vi "Recursive path search.vi"(6 "File name with extension":string, 8 "error in":errorcluster, 11 "Path":path) -> (0 "error out":errorcluster, 3 "Path out":path)   [LabVIEW 2019, in "TDMS.lvlib" / "TDMS.lvclass"]
uses:
  TDMS.lvclass
  <vilib>/Utility/sysdir.llb/System Directory Type.ctl
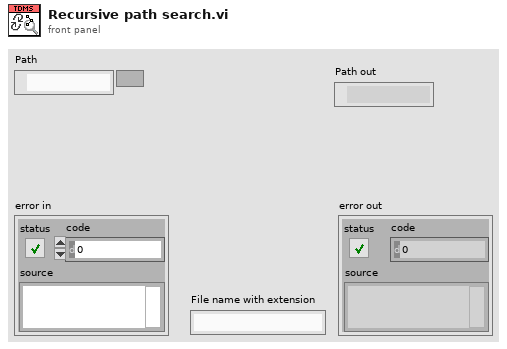
[diagram p1: front panel]
types:
  T1 = typedef "System Directory Type.ctl" = i32
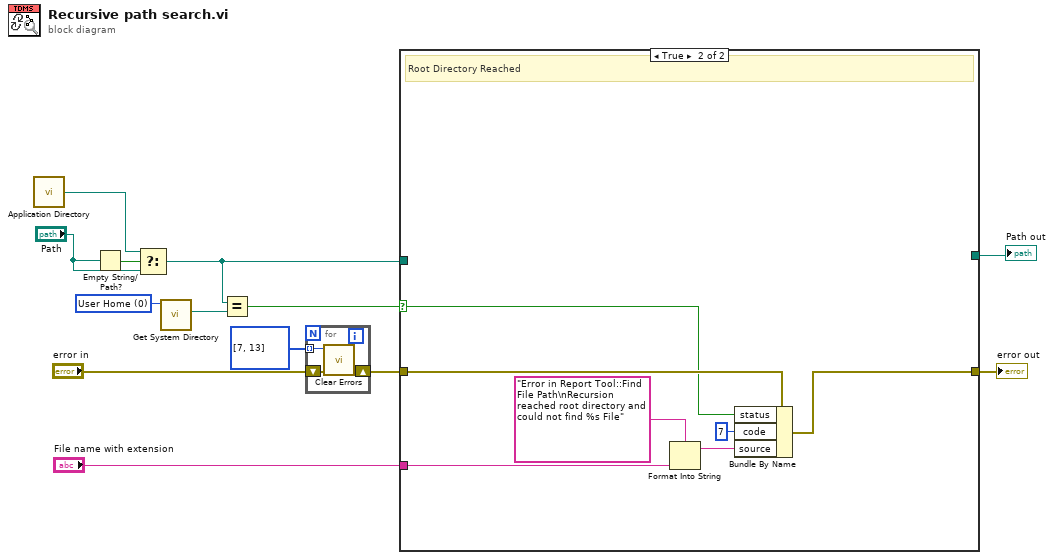
[diagram p0: block diagram]
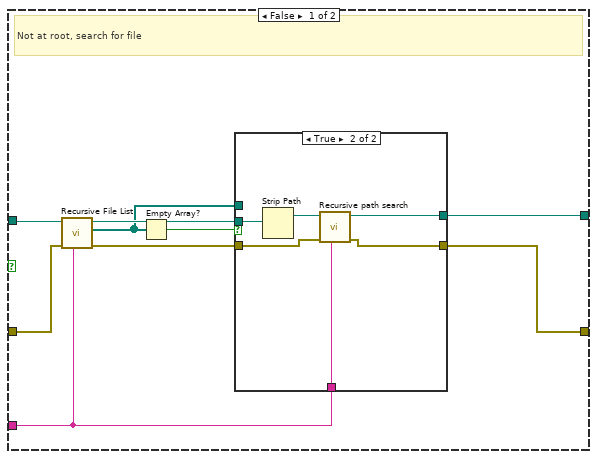
[diagram p2: hidden frame]
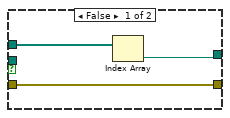
[diagram p3: hidden frame]
diagram:
  w9 = T1 0 items=["User Home"=0, "User Desktop"=1, "User Documents"=2, "User Application Data"=3, "User Preferences"=4, "User Temporary"=5, "Public Documents"=6, "Public Application Data"=7, "Public Preferences"=8, "Public Cache"=13, "System Core Libraries"=9, "System Installed Libraries"=10, "Application Files"=11, "Boot Volume Root"=12] ("system directory type")
  n1 = call <vilib>:"Application Directory.vi"() -> ("Application Directory"=w10:path)
  n2 = Empty String/Path?(string/path="Path") -> (empty?=w12:bool)
  n3 = Select(t=w10, s=w12, f="Path") -> (s? t:f=w3:path)
  n4 = call <vilib>:"Get System Directory.vi"("system directory type"=w9) -> ("system directory"=w8:path)  [unwired: 10 in]
  n5 = Equal?(x=w3, y=w8) -> (x = y?=w5:bool)
  n6 = for {
    tunnel: i32[] [7, 13] -> [w16] mode=indexing
    shift-right: [w15] -> w6
    shift-left: "error in" -> [w14]
    n7 = call <vilib>:"Clear Errors.vi"("error in (no error)"=w14, "specific error code to clear (0: all)"=w16) -> ("error out"=w15:errorcluster)  [unwired: 4 in, 1 out]
  }
  n8 = case shown="True" w5 {
    selector: w5 -> [_ w40]
    tunnel: w6 -> [w24 w41]
    tunnel: "File name with extension" -> [w21 w36]
    tunnel: w3 -> [w25 _]
    tunnel: [w20 _] -> w2
    tunnel: [w17 w35] -> w1
    frame False {
      # "Not at root, search for file"
      n9 = call <vilib>:"Recursive File List.vi"("pattern"=w21, "error in (no error)"=w24, "Folder Path"=w25) -> ("error out"=w19:errorcluster, "All Files in Dir"=w18:path[], "dup Folder Path"=w22:path)  [unwired: 4 in, 2 out]
      n10 = Empty Array?(array=w18) -> (empty?=w23:bool)
      n11 = case shown="True" w23 {
        tunnel: w22 -> [_ w34]
        tunnel: w21 -> [_ w33]
        tunnel: [w27 w31] -> w20
        tunnel: w19 -> [w26 w30]
        tunnel: w18 -> [w28 _]
        tunnel: [w26 w29] -> w17
        frame False {
          n12 = Index Array(array=w28) -> (element=w27:path)  [unwired: 1 in]
        }
        frame True {
          n13 = Strip Path(path=w34) -> (stripped path=w32:path)  [unwired: 1 out]
          n14 = call "Recursive path search.vi"("File name with extension"=w33, "error in"=w30, "Path"=w32) -> ("error out"=w29:errorcluster, "Path out"=w31:path)  [unwired: 7 in]
        }
      }
    }
    frame True {
      # "Root Directory Reached"
      n15 = Format Into String(format string="Error in Report Tool::Find File Path\nRecursion reached root directory and could not find %s File" ("source"), w36) -> (resulting string=w38:string)  [unwired: 2 in, 1 out]
      n16 = Bundle By Name(cluster=w41, "status"=w40, "code"=7, "source"=w38) -> (w35:errorcluster)
    }
  }
  "Path out" <- w2
  "error out" <- w1
